vi "StatusLEDFlash.vi"(8 "Error In":errorcluster, 9 "LINX Resource in":T1, 10 "DO Channel":u8, 11 "Boolean in":refnum<vi>) -> (0 "Error Out":errorcluster, 3 "LINX Resource out":T1)   [LabVIEW 2014]
uses:
  <vilib>/MakerHub/LINX/Private/Type Defs/LINX Ref.ctl
  <vilib>/MakerHub/LINX/Private/Type Defs/Platform.ctl
  <vilib>/MakerHub/LINX/Private/Type Defs/Interface.ctl
  <vilib>/MakerHub/LINX/Private/Device/Type Defs/LINX Device Config.ctl
  <vilib>/MakerHub/LINX/Private/Device/Type Defs/TCP Config.ctl
  <vilib>/MakerHub/LINX/Private/Device/Type Defs/Channels.ctl
  <vilib>/MakerHub/LINX/Public/Peripherals/Digital/Digital Write 1 Chan.vi
  <vilib>/MakerHub/LINX/Public/Peripherals/Digital/Digital Write N Chans.vi
  <vilib>/MakerHub/LINX/Private/Local IO/LinxDigitalWrite.vi
  <vilib>/MakerHub/LINX/Public/Utilities/Check Channel.vi
  <vilib>/MakerHub/LINX/Private/Local IO/Handle Errors.vi
  <vilib>/MakerHub/LINX/Private/Utilties/Generate Error.vi
  <vilib>/MakerHub/LINX/LMH-LINX.lvlib
  <vilib>/MakerHub/LINX/Private/Device/Device.lvlib
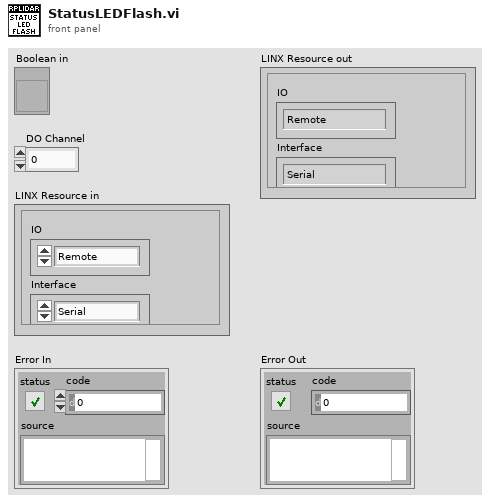
[diagram p1: front panel]
types:
  T1 = typedef "LMH-LINX.lvlib/LINX Ref.ctl" = cluster{"IO":T2, "Interface":T3, "LINX Device Config":T4}
  T2 = typedef "LMH-LINX.lvlib/Platform.ctl" = enum16{"Remote", "Local"}
  T3 = typedef "LMH-LINX.lvlib/Interface.ctl" = enum16{"Serial", "TCP"}
  T4 = typedef "LMH-LINX.lvlib/Device.lvlib/LINX Device Config.ctl" = cluster{"Interface":T3, "COM Port":refnum<visa-resource-name>, "TCP Configuration":T5, "Device Family":u8, "Device ID":u8, "Device Name":string, "TCP Ref":refnum<k5>, "Channels":T6}
  T5 = typedef "LMH-LINX.lvlib/Device.lvlib/TCP Config.ctl" = cluster{"IP Address":string, "Port":u16}
  T6 = typedef "LMH-LINX.lvlib/Channels.ctl" = cluster{"DI":u8[], "DO":u8[], "AI":u8[], "AO":u8[], "PWM":u8[], "QE":u8[], "UART":u8[], "I2C 2":u8[], "SPI":u8[], "CAN":u8[], "Servo":u8[], "AI Ref (V)":dbl, "AI Resolution (Bits)":u8, "AO Ref (V)":dbl, "AO Resolution (Bits)":u8}
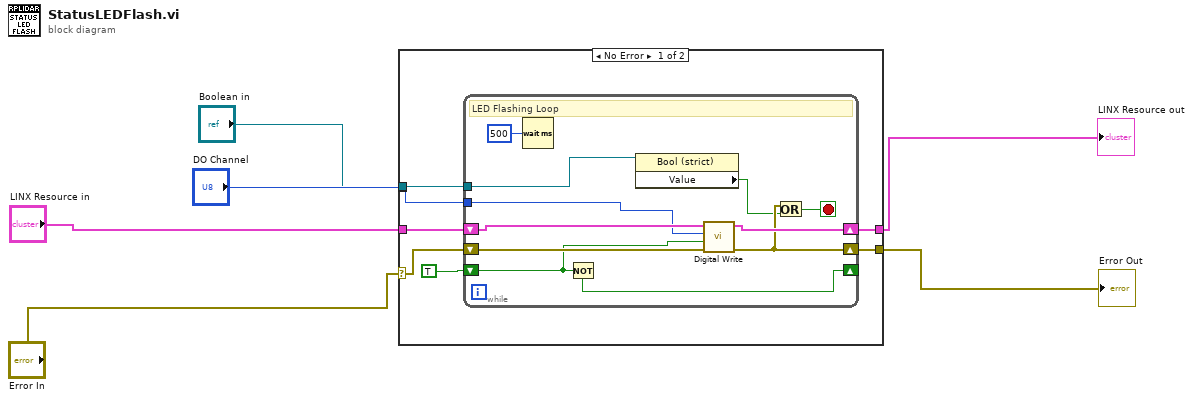
[diagram p0: block diagram]
diagram:
  n1 = case shown="No Error" "Error In" {
    selector: "Error In" -> [w7 w25]
    tunnel: "DO Channel" -> [w13 _]
    tunnel: [w12 w25] -> w5
    tunnel: "LINX Resource in" -> [w11 w26]
    tunnel: [w10 w26] -> w3
    tunnel: "Boolean in" -> [w8 _]
    frame No Error {
      n2 = while {
        shift-right: [w23] -> w10
        shift-left: w11 -> [w24]
        shift-right: [w21] -> w12
        shift-left: w7 -> [w22]
        shift-right: [w19] -> _
        shift-left: TRUE -> [w18]
        tunnel: w13 -> [w15]
        tunnel: w8 -> [w14]
        stop <- w17 stop-if-true
        # "LED Flashing Loop"
        n3 = Wait (ms)(milliseconds to wait=u32 500) -> ()  [unwired: 1 out]
        n4 = Not(x=w18) -> (.not. x?=w19:bool)
        n5 = property class="Bool (strict)"(reference=w14) -> ("Value"=w16:bool)  [unwired: 1 in, 2 out]
        n6 = call-poly <vilib>:"Digital Write.vi"("Error In"=w22, "Output Value"=w18, "DO Channel"=w15, "LINX Resource"=w24) -> ("Error Out"=w21:errorcluster, "LINX Resource"=w23:T1)  [unwired: 6 in]
        n7 = Or(x=w21, y=w16) -> (x .or. y?=w17:bool)
      }
    }
    frame Error {
    }
  }
  "Error Out" <- w5
  "LINX Resource out" <- w3
